vi "optionsAcq_spectralRange_waveNr.vi"(0 "reference":refnum<class "OSA200.lvclass">, 1 "range min (waveNr)":sgl, 2 "range max (waveNr)":sgl, 3 "write action":enum16{"range min", "range max", "both"}(ring), 4 "readWrite":enum16{"read", "write"}(ring), 5 "error in (no error)":errorcluster) -> (14 "duplicate reference":refnum<class "OSA200.lvclass">, 15 "range min read (waveNr)":sgl, 16 "range max read (waveNr)":sgl, 19 "error out":errorcluster)   [LabVIEW 2010, in "OSA200.lvclass"]
doc: "optionsAcq_spectralRange_waveNr enables a reduction of the spectrum dataset size while maintaining resolution. This is done by calling the functions 'FTS_SetAcquisitionOption_MinWaveNr' and 'FTS_SetAcquisitionOption_MaxWaveNr' with the desired wavenumber range. \n\nNotice that this cutting is done during the calculation of the spectrum from the interferogram and does not affect the interferogram at all, nor the time required to perform a measurement, (spectra update time unchanged).\n\nA smaller spectrum dataset can also be obtained by switching to low resolution mode. \n\nIn write mode; the spectrum graph x range will be updated accordingly, (plot_spectrum.vi will update graph with new range). This applies to spectrum graph which reference has been wired to init.vi., (see tree.vi for compatible graph).\n\nIn write both mode; the range min and max will be swapped if min being larger than max."
uses:
  OSA200.lvclass
  OSA.lvclass
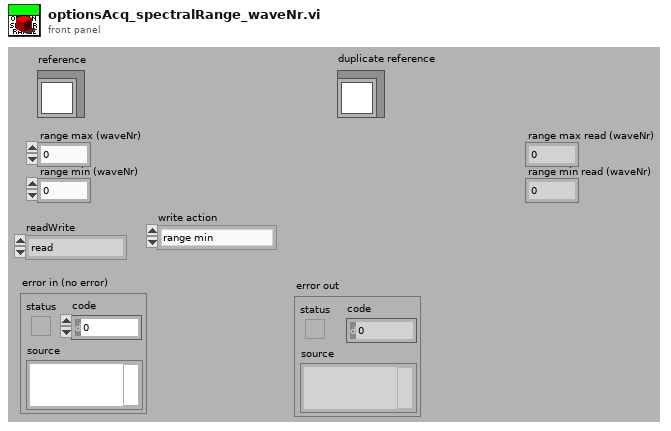
[diagram p1: front panel]
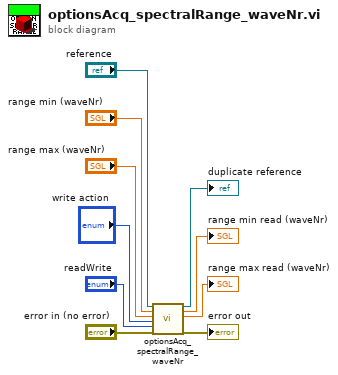
[diagram p0: block diagram]
diagram:
  n1 = call-parent "optionsAcq_spectralRange_waveNr.vi"("reference"="reference", "range min (waveNr)"="range min (waveNr)", "range max (waveNr)"="range max (waveNr)", "write action"="write action", "readWrite"="readWrite", "error in (no error)"="error in (no error)") -> ("duplicate reference"=→"duplicate reference":refnum<class "OSA200.lvclass">, "range min read (waveNr)"=→"range min read (waveNr)":sgl, "range max read (waveNr)"=→"range max read (waveNr)":sgl, "error out"=→"error out":errorcluster)  [unwired: 10 in]
